vi "Post Result.vi"(8 "error in (no error)":errorcluster, 10 "Results Notifier":refnum<notifier>, 11 "ReadCommand in":refnum<class "ReadCommand.lvclass">) -> (0 "error out":errorcluster, 3 "ReadCommand out":refnum<class "ReadCommand.lvclass">)   [LabVIEW 2023, in "HAF.lvlib" / "ReadCommand.lvclass"]
doc: "Posts the Result (complete Command with Raw Result set) onto the Notification Queue so that clients can pick it up and Process it."
uses:
  ReadCommand.lvclass
  All Notification Message Ids.ctl
  Global Resources.vi
  HAF.lvlib
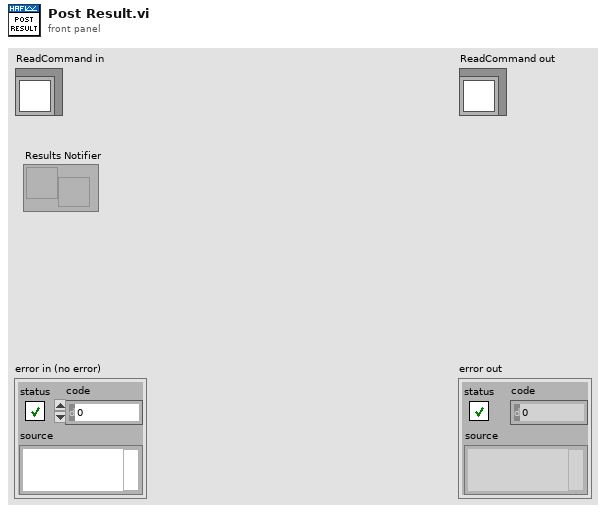
[diagram p1: front panel]
types:
  T1 = typedef "HAF.lvlib/All Notification Message Ids.ctl" = cluster{"Initialise":string, "Exit":string, "Error":string, "Result":string, "Done":string}
  T2 = typedef "HAF.lvlib/All Message Queues.ctl" = cluster{"Internal":refnum<queue>, "Notifications":refnum<queue>}
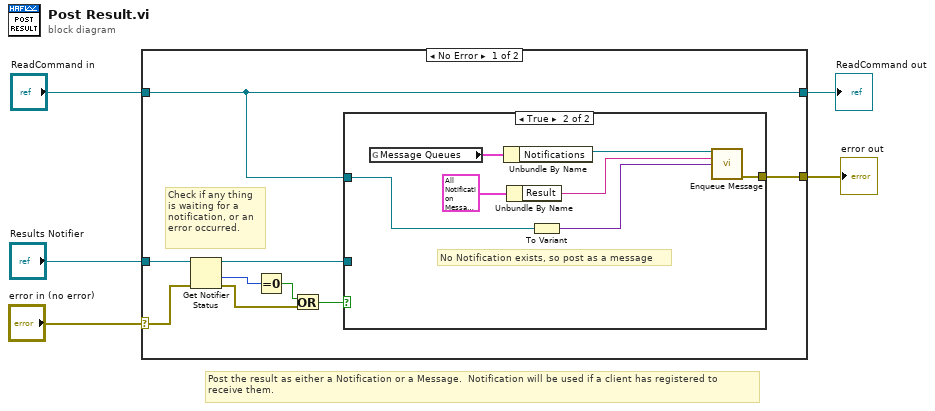
[diagram p0: block diagram]
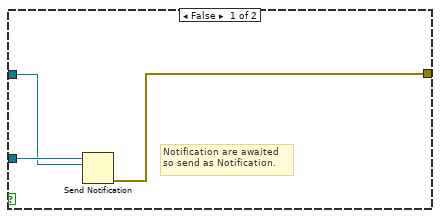
[diagram p2: hidden frame]
diagram:
  # "Post the result as either a Notification or a Message.  Notification will be used if a client has registered to \nreceive them."
  n1 = case shown="No Error" "error in (no error)" {
    selector: "error in (no error)" -> [w13 w26]
    tunnel: [w7 w26] -> w4
    tunnel: [w6 w25] -> w2
    tunnel: "ReadCommand in" -> [w6 w25]
    tunnel: "Results Notifier" -> [w14 _]
    frame No Error {
      # "Check if any thing\nis waiting for a \nnotification, or an\nerror occurred."
      n2 = Get Notifier Status(notifier=w14, error in (no error)=w13) -> (notifier out=w8:refnum<notifier>, # waiting=w12:i32, error out=w10:errorcluster)  [unwired: 2 out]
      n3 = Equal To 0?(x=w12) -> (x = 0?=w11:bool)
      n4 = Or(x=w11, y=w10) -> (x .or. y?=w9:bool)
      n5 = case shown="True" w9 {
        tunnel: w8 -> [w17 _]
        tunnel: w6 -> [w16 w20]
        tunnel: [w15 w18] -> w7
        frame False {
          # "Notification are awaited \nso send as Notification."
          n6 = Send Notification(notification=w16, notifier=w17) -> (error out=w15:errorcluster)  [unwired: 1 in, 1 out]
        }
        frame True {
          # "No Notification exists, so post as a message"
          n7 = global read "Global Resources.vi" "Message Queues"() -> (w24:T2)
          n8 = Unbundle By Name(w24) -> ("Notifications"=w22:refnum<queue>)
          n9 = Unbundle By Name(T1 {"Initialise"="Initialise", "Exit"="Exit", "Error"="Error", "Result"="Result", "Done"="Done"} ("Message IDs")) -> ("Result"=w21:string)
          n10 = To Variant(anything=w20) -> (Variant=w19:variant)
          n11 = call "Enqueue Message.vi"("Message Queue In"=w22, "Message Id"=w21, "Message Data"=w19) -> ("error out"=w18:errorcluster)  [unwired: 11 in, 1 out]
        }
      }
    }
    frame Error {
    }
  }
  "error out" <- w4
  "ReadCommand out" <- w2
